vi "HumanExecuteOutreach.vi"(8 "error in (no error)":errorcluster) -> (0 "error out":errorcluster)   [LabVIEW 2023]
doc: "Execute for Human\n\ninput:\n error in (cluster)\n\noutput:\n error out (cluster)"
uses:
  <vilib>/Rock Robotics/WPI/Joystick/XBox Buttons Indexer.ctl
  <vilib>/Rock Robotics/WPI/Joystick/XBox Axes Indexer.ctl
  <vilib>/Rock Robotics/WPI/ThirdParty/JAS_Junk/TrajLib/VI/BoolCmd_Send_Internal.vi
  <vilib>/Rock Robotics/WPI/ThirdParty/JAS_Junk/TrajLib/VI/BoolCmd_ObtainQueue.vi
  <vilib>/Rock Robotics/Network Tables/NT Write String.vi
  <vilib>/Rock Robotics/WPI/ThirdParty/JAS_Junk/TrajLib/Trajectory_Library.lvlib
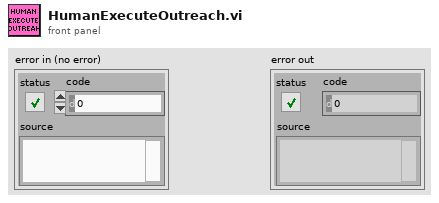
[diagram p1: front panel]
types:
  T1 = typedef "XBox Buttons Indexer.ctl" = enum16{"A", "B", "X", "Y", "Left Bumper", "Right Bumper", "Back", "Start", "Left Joystick", "Right Joystick"}
  T2 = typedef "XBox Axes Indexer.ctl" = enum16{"Left X", "Left Y", "Left Trigger", "Right Trigger", "Right X", "Right Y"}
  T3 = typedef "WPI_JoystickDevRef.ctl" = cluster{"Device":T4}
  T4 = typedef "WPI_JoystickDeviceEnum.ctl" = enum16{"USB 0", "USB 1", "USB 2", "USB 3", "USB 4", "USB 5"}
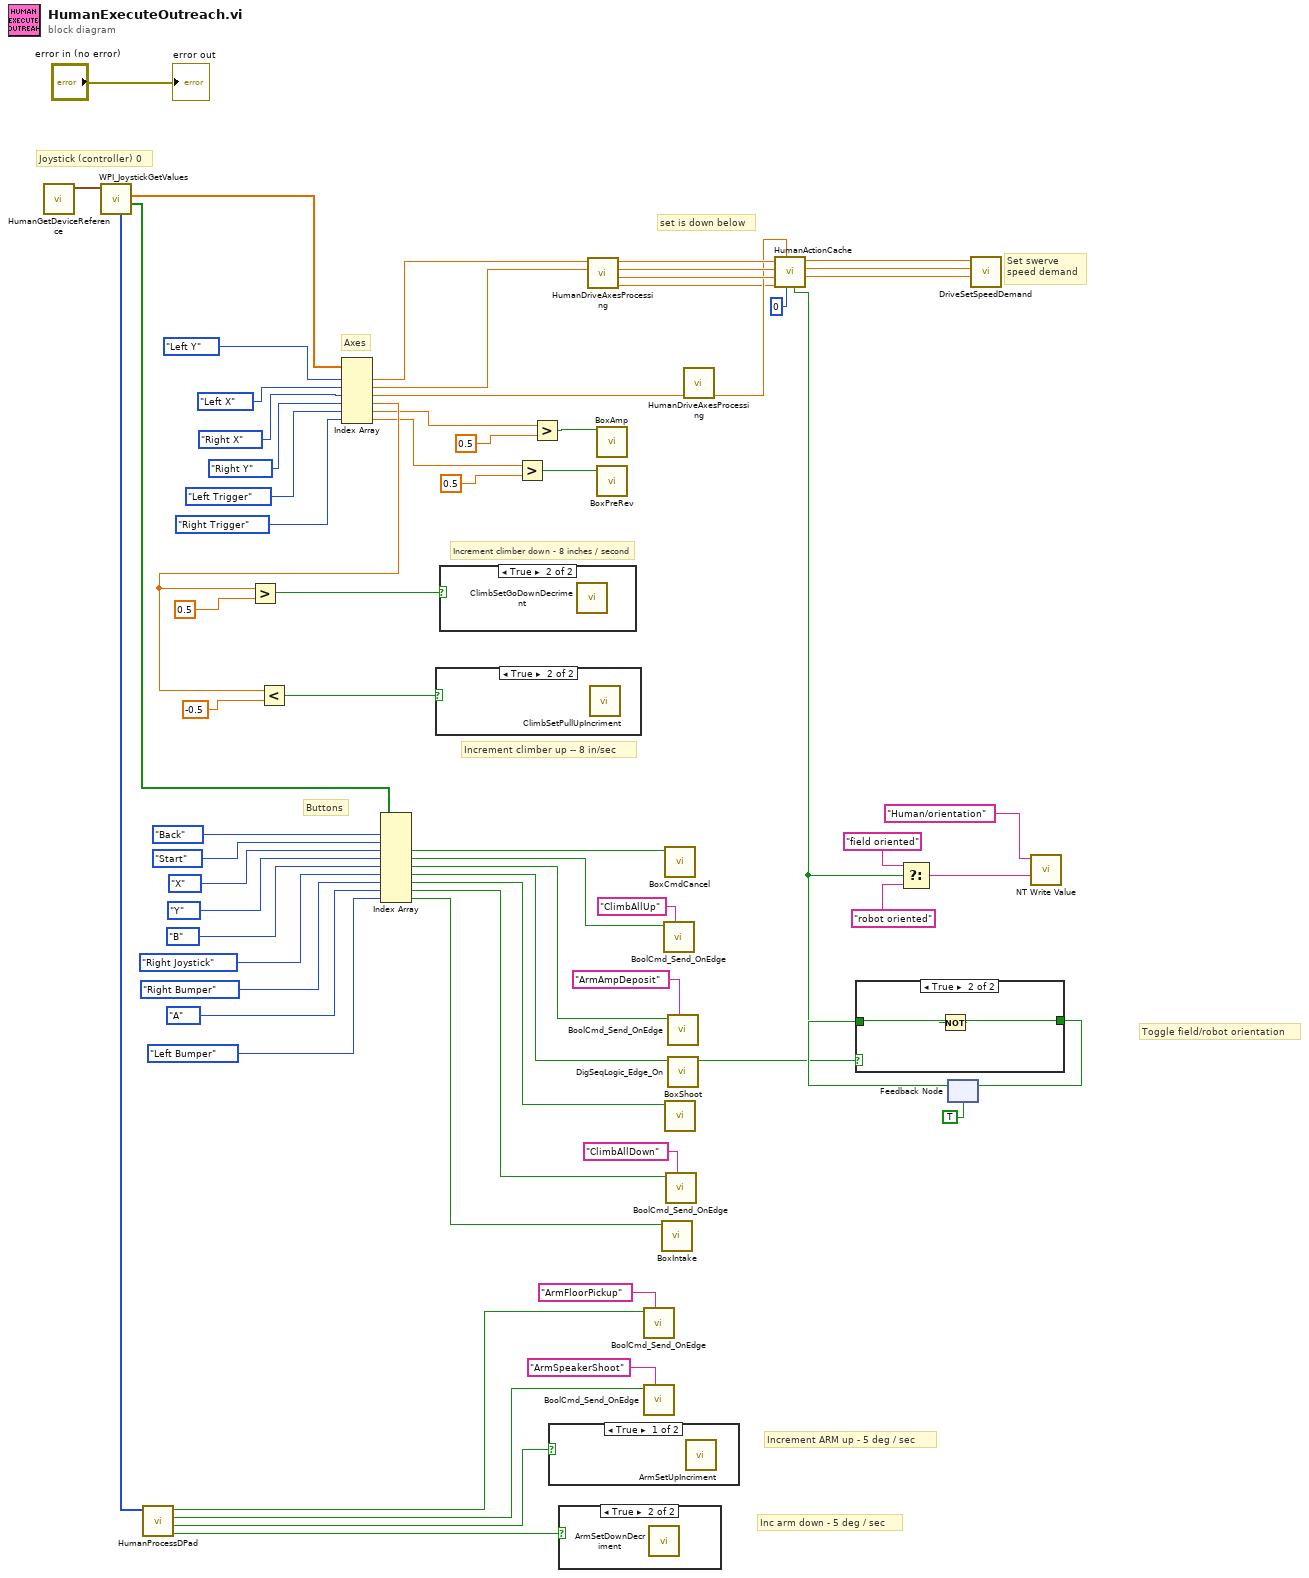
[diagram p0: block diagram]
diagram:
  # "Increment ARM up - 5 deg / sec"
  # "Inc arm down - 5 deg / sec"
  # "Increment climber up -- 8 in/sec"
  # "Increment climber down - 8 inches / second"
  # "Toggle field/robot orientation"
  # "Buttons"
  # "Axes"
  # "set is down below"
  # "Set swerve\nspeed demand"
  # "Joystick (controller) 0"
  n1 = call "HumanGetDeviceReference.vi"() -> ("Driver Joy"=w57:T3)  [unwired: 9 in, 2 out]
  n2 = call <vilib>:"WPI_JoystickGetValues.vi"("JoystickDevRef"=w57) -> ("Buttons"=w55:bool[], "Axes"=w56:dbl[], "POVs"=w66:i16[])  [unwired: 6 in, 2 out]
  n3 = call "HumanProcessDPad.vi"("POV"=w66) -> ("Right"=w17:bool, "Left"=w16:bool, "Down"=w12:bool, "Up"=w14:bool)  [unwired: 7 in]
  n4 = Index Array(array=w56, index #1=XBox_Axes_Indexer."Left Y" ("XBox Axes"), index #2=XBox_Axes_Indexer."Left X" ("XBox Axes"), index #3=XBox_Axes_Indexer."Right X" ("XBox Axes"), index #4=XBox_Axes_Indexer."Right Y" ("XBox Axes"), index #5=XBox_Axes_Indexer."Left Trigger" ("XBox Axes"), index #6=XBox_Axes_Indexer."Right Trigger" ("XBox Axes")) -> (element #1=w65:dbl, element #2=w64:dbl, element #3=w1:dbl, element #4=w28:dbl, element #5=w8:dbl, element #6=w7:dbl)
  n5 = Greater?(x=w28, y=0.5) -> (0:w29:bool)
  n6 = Less?(x=w28, y=-0.5) -> (x < y?=w30:bool)
  n7 = Index Array(array=w55, index #1=XBox_Buttons_Indexer."Back" ("Nothing"), index #2=XBox_Buttons_Indexer."Start" ("Nothing"), index #3=XBox_Buttons_Indexer."X" ("Nothing"), index #4=XBox_Buttons_Indexer."Y" ("Nothing"), index #5=XBox_Buttons_Indexer."B" ("Nothing"), index #6=XBox_Buttons_Indexer."Right Joystick" ("Nothing"), index #7=XBox_Buttons_Indexer."Right Bumper" ("Nothing"), index #8=XBox_Buttons_Indexer."A" ("Nothing"), index #9=XBox_Buttons_Indexer."Left Bumper" ("Nothing")) -> (element #3=w25:bool, element #4=w26:bool, element #5=w20:bool, element #6=w48:bool, element #7=w4:bool, element #8=w22:bool, element #9=w5:bool)  [unwired: 2 out]
  n8 = case shown="True" w30 {
    frame False {
    }
    frame True {
      n9 = call "ClimbSetPullUpIncriment.vi"() -> ()  [unwired: 11 in, 1 out]
    }
  }
  n10 = case shown="True" w29 {
    frame False {
    }
    frame True {
      n11 = call "ClimbSetGoDownDecriment.vi"() -> ()  [unwired: 11 in, 1 out]
    }
  }
  n12 = Greater?(x=w7, y=0.5) -> (0:w3:bool)
  n13 = Greater?(x=w8, y=0.5) -> (0:w6:bool)
  n14 = case shown="True" w16 {
    frame True {
      n15 = call "ArmSetUpIncriment.vi"() -> ()  [unwired: 11 in, 1 out]
    }
    frame False {
    }
  }
  n16 = case shown="True" w17 {
    frame False {
    }
    frame True {
      n17 = call "ArmSetDownDecriment.vi"() -> ()  [unwired: 11 in, 1 out]
    }
  }
  n18 = call "HumanDriveAxesProcessing.vi"("Left X"=w64, "Left Y"=w65) -> ("Right X"=w37:dbl, "Right Y"=w62:dbl, "Left X"=w63:dbl, "Left Y"=w61:dbl)  [unwired: 6 in]
  n19 = call "BoxAmp.vi"("box amp"=w6) -> ()  [unwired: 11 in]
  n20 = call "BoxPreRev.vi"("PreRev"=w3) -> ()  [unwired: 10 in, 1 out]
  n21 = call <vilib>:"BoolCmd_Send_OnEdge.vi"("Command Name"="ArmFloorPickup", "Value"=w14) -> ()  [unwired: 9 in, 1 out]
  n22 = call <vilib>:"BoolCmd_Send_OnEdge.vi"("Command Name"="ArmSpeakerShoot", "Value"=w12) -> ()  [unwired: 9 in, 1 out]
  n23 = call "BoxIntake.vi"("Box intake"=w5) -> ()  [unwired: 10 in, 1 out]
  n24 = call <vilib>:"BoolCmd_Send_OnEdge.vi"("Command Name"="ClimbAllUp", "Value"=w26) -> ()  [unwired: 9 in, 1 out]
  n25 = call "BoxCmdCancel.vi"("box cancel"=w25) -> ()  [unwired: 11 in]
  n26 = call "BoxShoot.vi"("Box shoot"=w4) -> ()  [unwired: 10 in, 1 out]
  n27 = call <vilib>:"BoolCmd_Send_OnEdge.vi"("Command Name"="ClimbAllDown", "Value"=w22) -> ()  [unwired: 9 in, 1 out]
  n28 = call <vilib>:"BoolCmd_Send_OnEdge.vi"("Command Name"="ArmAmpDeposit", "Value"=w20) -> ()  [unwired: 9 in, 1 out]
  n29 = call <vilib>:"DigSeqLogic_Edge_On.vi"("Input"=w48) -> ("On Edge"=w46:bool)  [unwired: 10 in]
  n30 = call "HumanDriveAxesProcessing.vi"("Right X"=w1) -> ("Right X"=w38:dbl)  [unwired: 7 in, 3 out]
  n31 = feedback #1(TRUE) -> (w47:bool)
  n32 = case shown="True" w46 {
    tunnel: w47 -> [w68 w70]
    tunnel: [w68 w69] -> w44
    frame False {
    }
    frame True {
      n33 = Not(x=w70) -> (.not. x?=w69:bool)
    }
  }
  n34 = call "HumanActionCache.vi"("Enable Field Oriented Drive"=w44, "State"=0, "Rotation"=w38, "Right X"=w37, "Right Y"=w62, "Left X"=w63, "Left Y"=w61) -> ("AMotorDemand"=w60:dbl, "YMotorDemand"=w59:dbl, "XMotorDemand"=w58:dbl)  [unwired: 2 in]
  n35 = Select(t="field oriented", s=w44, f="robot oriented") -> (s? t:f=w41:string)
  n36 = feedback-in #1(w44) -> ()
  n37 = call "DriveSetSpeedDemand.vi"("ASpeedDemand (d/s)"=w60, "YSpeedDemand (ft/s)"=w59, "XSpeedDemand (ft/s)"=w58) -> ()  [unwired: 9 in]
  n38 = call-poly <vilib>:"NT Write Value.vi"("value"=w41, "name"="Human/orientation") -> ()  [unwired: 9 in, 1 out]
  "error out" <- "error in (no error)"
